vi "Set Self Cal.vi"(0 "shared in":refnum<class "niUSRP Rx Core v1 FPGA.lvclass">=refnum, 5 "self cal":refnum<class "Self Cal.lvclass">=refnum) -> (4 "shared out":refnum<class "niUSRP Rx Core v1 FPGA.lvclass">)   [LabVIEW 2023]
uses:
  <instrlib>/niUSRP/Reference FPGA/Rx Core/niUSRP Rx Core v1 FPGA.lvclass
  <instrlib>/niVST/Self Cal/v2/FPGA/Self Cal.lvclass
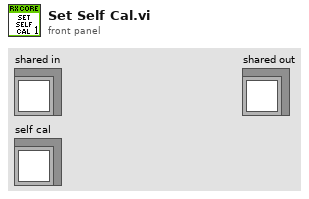
[diagram p1: front panel]
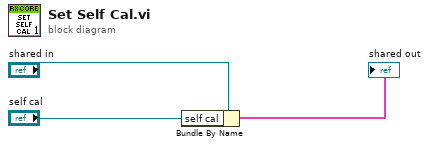
[diagram p0: block diagram]
diagram:
  n1 = Bundle By Name(cluster="shared in", "self cal"="self cal") -> (→"shared out":cluster{})
